vi "处理单按.vi"(0 "图片":picture, 5 "地图":dbl[][](array[numeric]), 7 "雷区":dbl[][](array[numeric]), 9 "行":dbl, 11 "列":dbl) -> (4 "图片 2":picture, 6 "地图 2":dbl[][](array[numeric]), 8 "是否踩雷":bool, 10 "是否合法":bool)   [LabVIEW 2023]
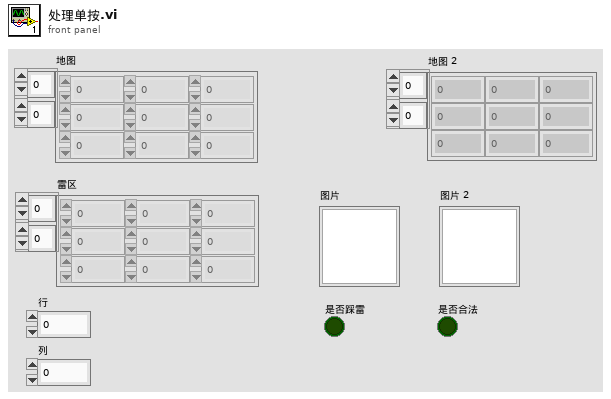
[diagram p1: front panel]
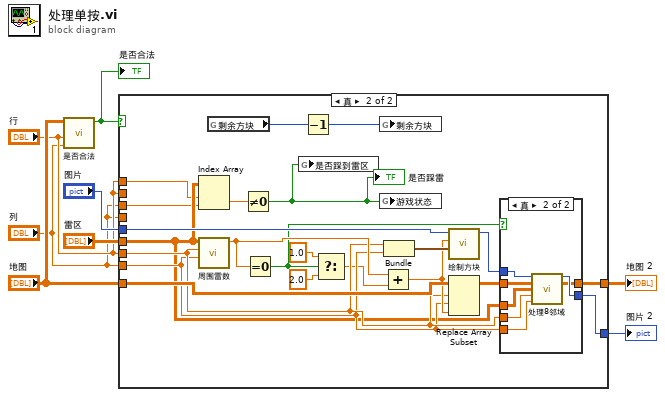
[diagram p0: block diagram]
diagram:
  n1 = call "是否合法.vi"("列"="列", "行"="行", "地图"="地图") -> ("是否合法"=w3:bool)  [unwired: 7 in, 1 out]
  "是否合法" <- w3
  n2 = case shown="真" w3 {
    tunnel: "雷区" -> [_ w18]
    tunnel: "地图" -> [w9 w31]
    tunnel: "行" -> [_ w23]
    tunnel: "列" -> [_ w22]
    tunnel: "图片" -> [w10 w32]
    tunnel: [w10 w21] -> w6
    tunnel: [w9 w20] -> w5
    tunnel: "行" -> [_ _]
    tunnel: "列" -> [_ _]
    tunnel: "行" -> [_ w17]
    tunnel: "列" -> [_ w16]
    frame False {
    }
    frame True {
      n3 = Index Array(array=w18, index (row)=w17, index (col)=w16) -> (element=w19:dbl)
      n4 = call "周围雷数.vi"("列"=w22, "行"=w23, "雷区"=w18) -> ("雷数"=w28:dbl)  [unwired: 8 in]
      n5 = global read "全局变量.vi" "剩余方块"() -> (w30:u16)
      n6 = Not Equal To 0?(x=w19) -> (x != 0?=w11:bool)
      "是否踩雷" <- w11
      n7 = Equal To 0?(x=w28) -> (x = 0?=w13:bool)
      n8 = global write "全局变量.vi" "是否踩到雷区"(w11) -> ()
      n9 = Decrement(x=w30) -> (x-1=w29:u16)
      n10 = Select(t=1.0, s=w13, f=2.0) -> (s? t:f=w12:dbl)
      n11 = global write "全局变量.vi" "剩余方块"(w29) -> ()
      n12 = global write "全局变量.vi" "游戏状态"(w11) -> ()
      n13 = Add(x=w28, y=w12) -> (x+y=w26:dbl)
      n14 = Bundle("行"=w23, "列"=w22) -> (w27:cluster{"行":dbl, "列":dbl})  [unwired: 1 in]
      n15 = call "绘制方块.vi"("簇"=w27, "ID"=w26, "picture"=w32) -> ("new picture"=w25:picture)  [unwired: 8 in]
      n16 = Replace Array Subset(array=w31, new element=w26, index (row)=w23, index (col)=w22) -> (w24:dbl[][])
      n17 = case shown="真" w13 {
        tunnel: w25 -> [w34 w41]
        tunnel: w24 -> [w33 w40]
        tunnel: w18 -> [_ w39]
        tunnel: w23 -> [_ w38]
        tunnel: w22 -> [_ w37]
        tunnel: [w34 w36] -> w21
        tunnel: [w33 w35] -> w20
        frame False {
        }
        frame True {
          n18 = call "处理8邻域.vi"("图片"=w41, "地图"=w40, "雷区"=w39, "行"=w38, "列"=w37) -> ("图片 2"=w36:picture, "地图 2"=w35:dbl[][])  [unwired: 9 in]
        }
      }
    }
  }
  "图片 2" <- w6
  "地图 2" <- w5
